vi "TIO RPC Send REQuest_Ser.vi"(8 "error in (no error)":errorcluster, 9 "Payload":string, 10 "Topic":string, 11 "Nom de ressource VISA":refnum<visa-resource-name>) -> (0 "error out":errorcluster, 2 "Request ID":u16=60741 format="%04x", 3 "Nom de ressource VISA Out":refnum<visa-resource-name>)   [LabVIEW 2010]
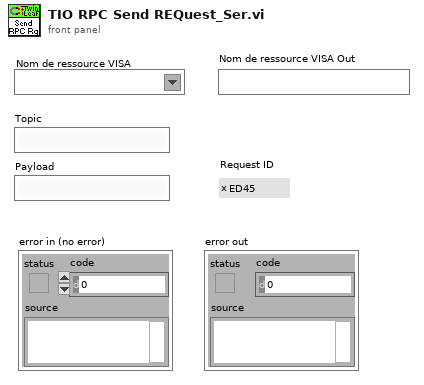
[diagram p1: front panel]
types:
  T1 = enum8{"Invalid", "Log", "RPC Request", "RPC Reply", "RPC Error", "Stream Description", "User"}
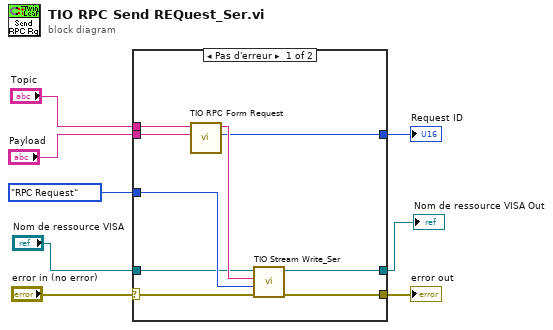
[diagram p0: block diagram]
diagram:
  n1 = case shown="Pas d'erreur" "error in (no error)" {
    selector: "error in (no error)" -> [w9 w19]
    tunnel: [w17 w19] -> w8
    tunnel: "Topic" -> [w16 _]
    tunnel: "Payload" -> [w15 _]
    tunnel: [w13 _] -> w5
    tunnel: T1."RPC Request" ("Type") -> [w12 _]
    tunnel: "Nom de ressource VISA" -> [w11 w18]
    tunnel: [w10 w18] -> w2
    frame No Error {
      n2 = call <userlib>:"TIO RPC Form Request.vi"("Payload"=w15, "Topic"=w16) -> ("Request ID"=w13:u16, "String out"=w14:string)  [unwired: 8 in]
      n3 = call <userlib>:"TIO Stream Write_Ser.vi"("error in (no error)"=w9, "Type"=w12, "Payload"=w14, "Nom de ressource VISA"=w11) -> ("error out"=w17:errorcluster, "Nom de ressource VISA Out"=w10:refnum<visa-resource-name>)  [unwired: 5 in]
    }
    frame Error {
    }
  }
  "error out" <- w8
  "Request ID" <- w5
  "Nom de ressource VISA Out" <- w2
